vi "practice.vi"() -> ()   [LabVIEW 2014]
uses:
  <vilib>/Utility/file.llb/Write To Spreadsheet File (DBL).vi
panel:
  out "XY Graph":cluster{"Time":dbl[], "Displacement":dbl[]}(graph)
  in  "AM Wave Parameters":T1
  in  "Digitizing Parameters":T2
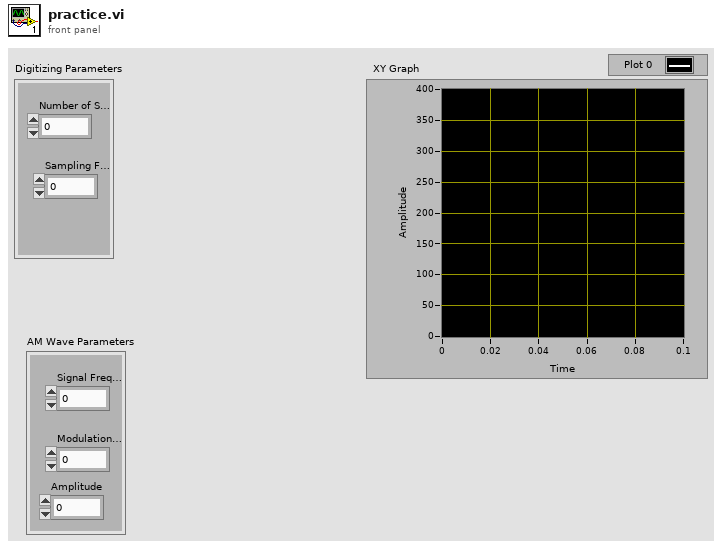
[diagram p1: front panel]
types:
  T1 = cluster{"Signal Frequency":dbl, "Modulation Frequency":dbl, "Amplitude":dbl}
  T2 = cluster{"Number of Samples":dbl, "Sampling Frequency":dbl}
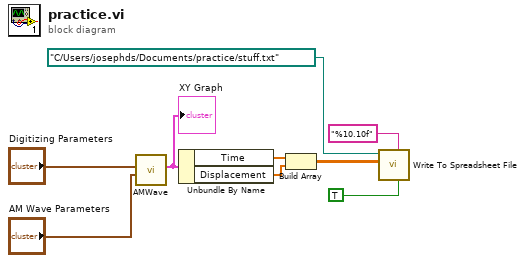
[diagram p0: block diagram]
diagram:
  n1 = call "AMWave.vi"("AM Wave Parameters"="AM Wave Parameters", "Digitizing Parameters"="Digitizing Parameters") -> ("output cluster"=w7:cluster{"Time":dbl[], "Displacement":dbl[]})  [unwired: 9 in]
  "XY Graph" <- w7
  n2 = Unbundle By Name(w7) -> ("Time"=w6:dbl[], "Displacement"=w5:dbl[])
  n3 = Build Array(w6, w5) -> (w4:dbl[][])
  n4 = call-poly <vilib>:"Write To Spreadsheet File.vi"("transpose? (no:F)"=TRUE, "format (%.3f)"="%10.10f", "2D data"=w4, "file path (dialog if empty)"=path "C:/Users/josephds/Documents/practice/stuff.txt") -> ()  [unwired: 4 in, 1 out]
